vi "StdDataPlot.vi"() -> (0 "Std Series":dbl[](array[numeric]) format="%#_11f", 3 "XY Graph":cluster{i32[], dbl[]}[](graph))   [LabVIEW 2023]
uses:
  <vilib>/Utility/file.llb/Read Delimited Spreadsheet (DBL).vi
panel:
  out "Array":i32[](array[numeric])
  out "x-1":i32
  out "Last":dbl format="%#_11f"
  out "Avr":dbl format="%#_4f"
  out "Size":i32
  in  "file path":path=path "/Users/blagojnikolov/Desktop/@tmp/sdtAllRes.txt"
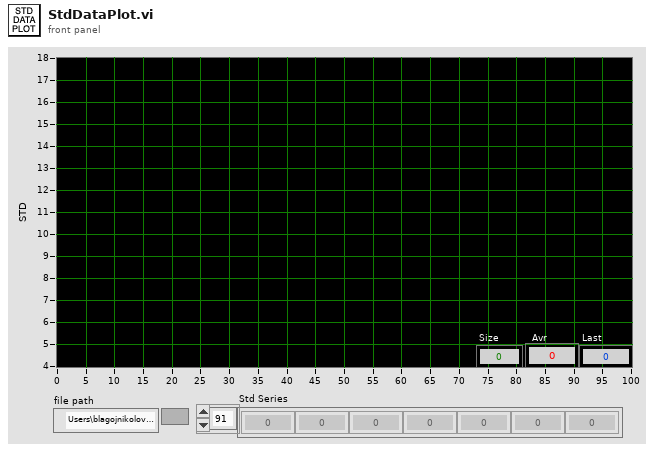
[diagram p1: front panel]
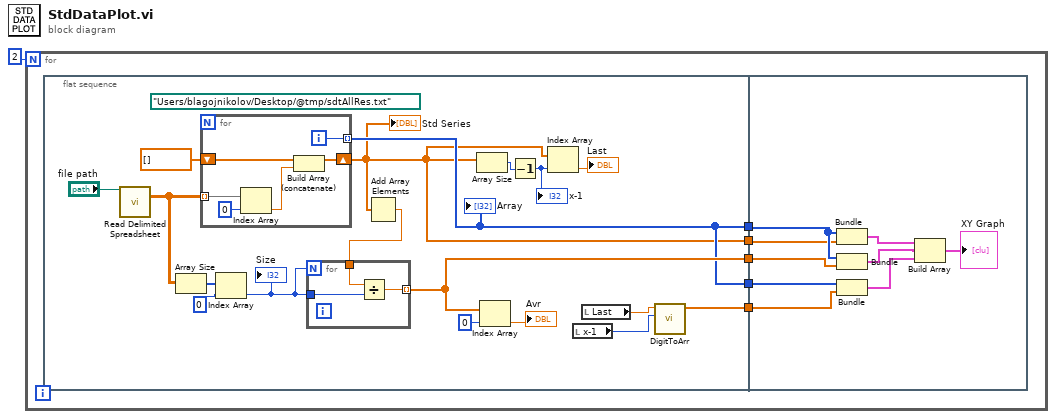
[diagram p0: block diagram]
diagram:
  n1 = for {
    N: 2 -> [_]
    n2 = flat-sequence {
      tunnel: [w18] -> w6
      tunnel: [w8] -> w5
      tunnel: [w9] -> w4
      tunnel: [w10] -> w3
      tunnel: [w9] -> w2
      tunnel: w6 -> [w37]
      tunnel: w5 -> [w36]
      tunnel: w4 -> [w38]
      tunnel: w3 -> [w35]
      tunnel: w2 -> [w34]
      frame #0 {
        (unwired) path "/Users/blagojnikolov/Desktop/@tmp/sdtAllRes.txt" ("file path 2")
        n3 = call-poly <vilib>:"Read Delimited Spreadsheet.vi"("file path (dialog if empty)"="file path") -> ("all rows"=w22:dbl[][])  [unwired: 9 in, 5 out]
        n4 = Array Size(array=w22) -> (size(s)=w21:i32[])
        n5 = for {
          tunnel: [w30] -> w9 mode=indexing
          tunnel: w22 -> [w32] mode=indexing
          shift-right: [w28] -> w8
          shift-left: dbl[] [] -> [w33]
          i -> [w30]
          n6 = Index Array "Index Array"(array=w32, index=0) -> (element=w31:dbl)
          n7 = Build Array (concatenate)(w33, w31) -> (w28:dbl[])
        }
        "Std Series" <- w8
        "Array" <- w9
        n8 = Index Array(array=w21, index=0) -> (element=w19:i32)
        "Size" <- w19
        n9 = Add Array Elements(numeric array=w8) -> (sum=w7:dbl)
        n10 = for {
          N: w19 -> [_]
          tunnel: [w25] -> w18 mode=indexing
          tunnel: w7 -> [w27]
          tunnel: w19 -> [w26]
          n11 = Divide(x=w27, y=w26) -> (x/y=w25:dbl)
        }
        n12 = Array Size(array=w8) -> (size(s)=w14:i32)
        n13 = Index Array(array=w18, index=0) -> (element=→"Avr":dbl)
        n14 = Decrement(x=w14) -> (x-1=w13:i32)
        "x-1" <- w13
        n15 = Index Array "Index Array"(array=w8, index=w13) -> (element=→"Last":dbl)
        n16 = local read "x-1"() -> (w12:i32)
        n17 = local read "Last"() -> (w11:dbl)
        n18 = call "DigitToArr.vi"("Arr Size"=w12, "Digit"=w11) -> ("Array out"=w10:dbl[])  [unwired: 9 in]
      }
      frame #1 {
        n19 = Bundle(w38, w36) -> (w39:cluster{i32[], dbl[]})  [unwired: 1 in]
        n20 = Bundle(w38, w37) -> (w40:cluster{i32[], dbl[]})  [unwired: 1 in]
        n21 = Bundle(w34, "Array out"=w35) -> (w42:cluster{i32[], "Array out":dbl[]})  [unwired: 1 in]
        n22 = Build Array(w39, w40, w42) -> (→"XY Graph":cluster{i32[], "Array out":dbl[]}[])
      }
    }
  }
